vi "Get ObjData.vi"(8 "error in (no error)":errorcluster, 11 "Application in":refnum<class "Application.lvclass">) -> (0 "error out":errorcluster, 2 "ObjData":T1, 3 "Application out":refnum<class "Application.lvclass">)   [LabVIEW 2019, in "Application.lvclass"]
doc: "Developed by Kevin Thompson\nkevin@thompsonengineering.net\n\nCopyright 2018\nThompson Engineering, LLC"
uses:
  Application.lvclass
  DataTypes/ObjData--cluster.ctl
  DataTypes/Read Data--cluster.ctl
  DataTypes/Settings--cluster.ctl
  Common/DataTypes/TD Async CmdMsg EventData--cluster.ctl
  DataTypes/Public Events--cluster.ctl
  DataTypes/Dependency--cluster.ctl
  <vilib>/TELLC/Dynamic CVT API/TD Dynamic CVT DVR--ref.ctl
  Subsystems/Main/Main.lvclass
  Subsystems/Config/Config.lvclass
  Common/ErrorHandler/ErrorHandler.lvclass
  Subsystems/DAQ_Engine/DAQ_Engine.lvclass
  Subsystems/Log_Engine/Log_Engine.lvclass
  Common/DataTypes/ChannelWaveforms--cluster.ctl
  Common/DataTypes/InverterWaveforms--cluster.ctl
  Common/DataTypes/InverterWaveforms--QRef.ctl
  Common/DataTypes/RawChannelData--cluster.ctl
  Common/DataTypes/RawDAQData--cluster.ctl
  Common/DataTypes/RawDAQDataQRef--cluster.ctl
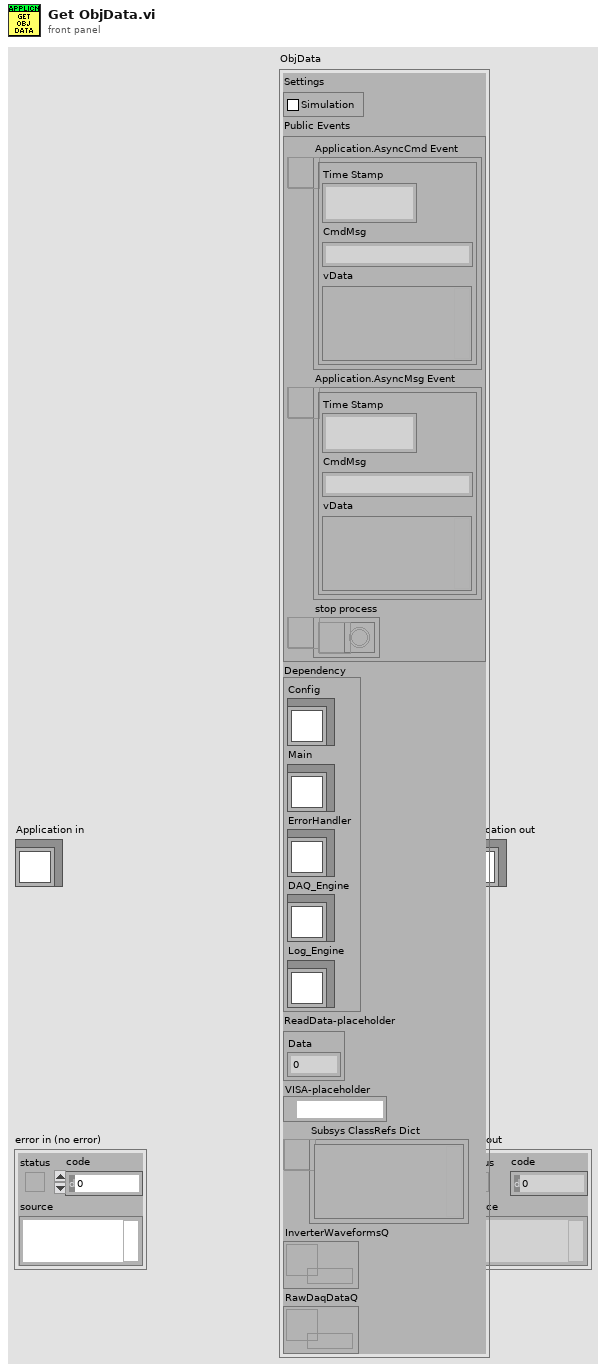
[diagram p1: front panel]
types:
  T1 = typedef "Application.lvclass/ObjData--cluster.ctl" = cluster{"Settings":T2, "Public Events":T3, "Dependency":T4, "ReadData-placeholder":T5, "VISA-placeholder":refnum<visa-resource-name>, "Subsys ClassRefs Dict":T6, "InverterWaveformsQ":T7, "RawDaqDataQ":T8}
  T2 = typedef "Application.lvclass/Settings--cluster.ctl" = cluster{"Simulation":bool}
  T3 = typedef "Application.lvclass/Public Events--cluster.ctl" = cluster{"Application.AsyncCmd Event":refnum<user-event>, "Application.AsyncMsg Event":refnum<user-event>, "stop process":refnum<user-event>}
  T4 = typedef "Application.lvclass/Dependency--cluster.ctl" = cluster{"Config":refnum<class "Config.lvclass">, "Main":refnum<class "Main.lvclass">, "ErrorHandler":refnum<class "ErrorHandler.lvclass">, "DAQ_Engine":refnum<class "DAQ_Engine.lvclass">, "Log_Engine":refnum<class "Log_Engine.lvclass">}
  T5 = typedef "Application.lvclass/Read Data--cluster.ctl" = cluster{"Data":dbl}
  T6 = typedef "TD Dynamic CVT DVR--ref.ctl" = refnum<data-value>
  T7 = typedef "InverterWaveforms--QRef.ctl" = refnum<queue>
  T8 = typedef "RawDAQDataQRef--cluster.ctl" = refnum<queue>
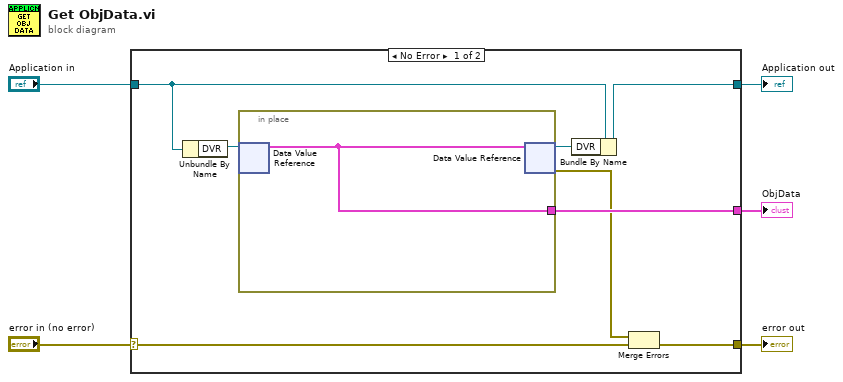
[diagram p0: block diagram]
diagram:
  n1 = case shown="No Error" "error in (no error)" {
    selector: "error in (no error)" -> [w13 w15]
    tunnel: [w7 w15] -> w4
    tunnel: [w9 w16] -> w2
    tunnel: "Application in" -> [w10 w16]
    tunnel: [w8 _] -> w1
    frame No Error {
      n2 = Unbundle By Name(w10) -> ("DVR"=w11:refnum<data-value>)
      n3 = in-place {
        in-place-border: [w14] -> w8
        n4 = in-place-dvr #1(w11) -> (w14:T1)  [unwired: 1 out]
        n5 = in-place-dvr #1(w14) -> (w12:refnum<data-value>, w6:errorcluster)
      }
      n6 = Bundle By Name(cluster=w10, "DVR"=w12) -> (w9:refnum<class "Application.lvclass">)
      n7 = Merge Errors(w6, w13) -> (w7:errorcluster)
    }
    frame Error {
    }
  }
  "error out" <- w4
  "Application out" <- w2
  "ObjData" <- w1
